vi "Framework.Get Cache.vi"(11 "Framework in":refnum<class "Framework.lvclass">) -> (2 "Cache":refnum<class "Cache.lvclass">, 3 "Framework out":refnum<class "Framework.lvclass">)   [LabVIEW 2017, in "DSF Core.lvlib" / "Framework.lvclass"]
uses:
  Framework.lvclass
  Cache/Cache.lvclass
  Framework.lvclass/Framework.ctl
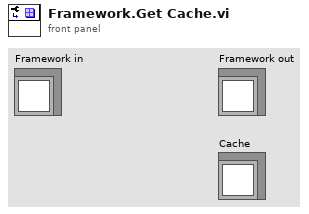
[diagram p1: front panel]
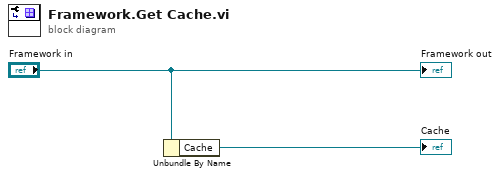
[diagram p0: block diagram]
diagram:
  n1 = Unbundle By Name("Framework in") -> ("Cache"=→"Cache":refnum<class "Cache.lvclass">)
  "Framework out" <- "Framework in"
